vi "Configure Sweep.vi"(6 "Sweep Interval (10.42 µs)":dbl=1.042e-05 format="%#_8g", 7 "Sweep Coupling (0:DC)":u16(ring) items=["DC", "AC"], 8 "error in (no error)":errorcluster, 9 "Sweep Points (0)":i32, 10 "Sweep Offset (0 Sec)":dbl, 11 "VISA resource name":refnum<visa-resource-name>) -> (0 "error out":errorcluster, 3 "VISA resource name out":refnum<visa-resource-name>)   [LabVIEW 2010, in "California Instruments iX Series.lvlib"]
doc: "Configures the measurement current range and the data acquire sequence of the AC source."
uses:
  <instrlib>/California Instruments iX Series/California Instruments iX Series.lvlib
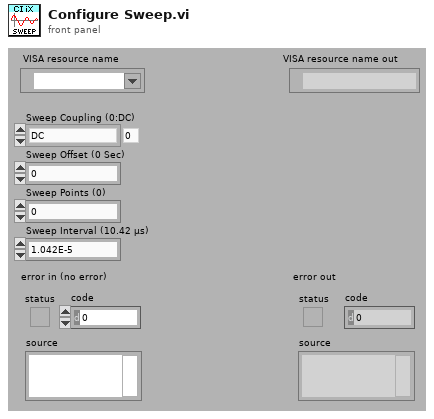
[diagram p1: front panel]
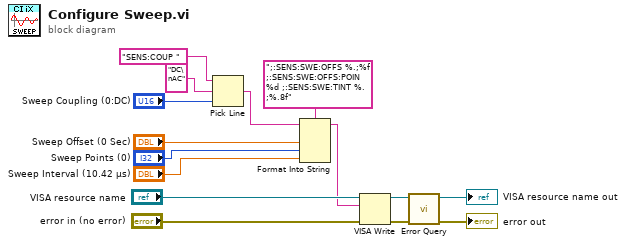
[diagram p0: block diagram]
diagram:
  n1 = Pick Line(string ("")="SENS:COUP ", multi-line string="DC\nAC", line index="Sweep Coupling (0:DC)") -> (output string=w3:string)
  n2 = Format Into String(format string=";:SENS:SWE:OFFS %.;%f ;:SENS:SWE:OFFS:POIN %d ;:SENS:SWE:TINT %.;%.8f", initial string=w3, "Sweep Offset (0 Sec)", "Sweep Points (0)", "Sweep Interval (10.42 µs)") -> (resulting string=w1:string)  [unwired: 1 in, 1 out]
  n3 = VISA Write(VISA resource name="VISA resource name", write buffer=w1, error in (no error)="error in (no error)") -> (VISA resource name out=w13:refnum<visa-resource-name>, error out=w12:errorcluster)  [unwired: 1 out]
  n4 = call <instrlib>:"Error Query.vi"("error in (no error)"=w12, "VISA resource name"=w13) -> ("error out"=→"error out":errorcluster, "VISA resource name out"=→"VISA resource name out":refnum<visa-resource-name>)  [unwired: 6 in, 2 out]
